vi "DecodePublicKey.vi"(3 "error in (no error) 2":errorcluster, 4 "Public Key":string) -> (0 "error out":errorcluster, 1 "e":cluster{"P/N":bool, "Array":u64[]}, 2 "n":cluster{"P/N":bool, "Array":u64[]})   [LabVIEW 2023]
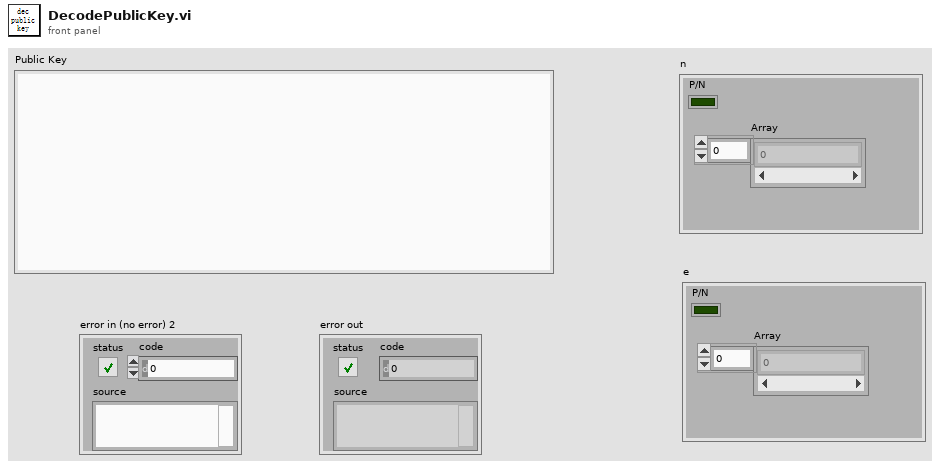
[diagram p1: front panel]
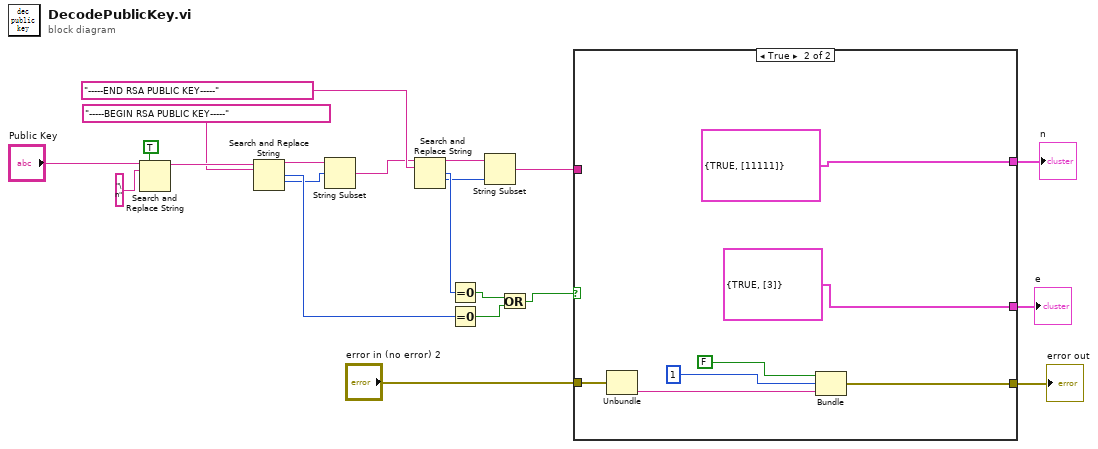
[diagram p0: block diagram]
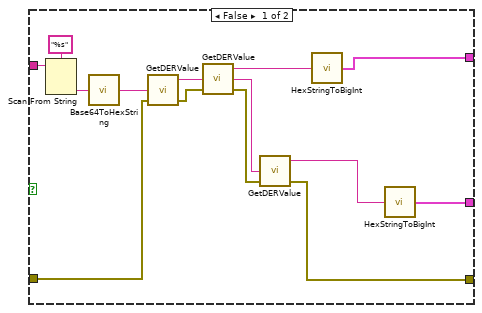
[diagram p2: hidden frame]
diagram:
  n1 = Search and Replace String(replace all?=TRUE, input string="Public Key", search string="\n") -> (result string=w18:string)  [unwired: 5 in, 3 out]
  n2 = Search and Replace String(input string=w18, search string="-----BEGIN RSA PUBLIC KEY-----") -> (result string=w13:string, number of replacements=w15:i32, offset past replacement=w12:i32)  [unwired: 6 in, 1 out]
  n3 = String Subset(string=w13, offset (0)=w12) -> (substring=w11:string)  [unwired: 1 in]
  n4 = Search and Replace String(input string=w11, search string="-----END RSA PUBLIC KEY-----") -> (result string=w10:string, number of replacements=w14:i32, offset past replacement=w9:i32)  [unwired: 6 in, 1 out]
  n5 = Equal To 0?(x=w14) -> (x = 0?=w7:bool)
  n6 = Equal To 0?(x=w15) -> (x = 0?=w6:bool)
  n7 = String Subset(string=w10, length (rest)=w9) -> (substring=w8:string)  [unwired: 1 in]
  n8 = Or(x=w7, y=w6) -> (x .or. y?=w5:bool)
  n9 = case shown="True" w5 {
    tunnel: w8 -> [w34 _]
    tunnel: [w29 cluster{bool, u64[]} {TRUE, [11111]}] -> w4
    tunnel: [w28 cluster{bool, u64[]} {TRUE, [3]}] -> w3
    tunnel: [w23 w36] -> w2
    tunnel: "error in (no error) 2" -> [w22 w40]
    frame False {
      n10 = Scan From String(format string="%s", input string=w34) -> (output 1=w33:string)  [unwired: 3 in, 3 out]
      n11 = call "Base64ToHexString.vi"("BASE64 string"=w33) -> ("Hex"=w31:string)
      n12 = call "GetDERValue.vi"("error in (no error)"=w22, "DER"=w31) -> ("error out"=w25:errorcluster, "value"=w30:string)  [unwired: 1 in, 1 out]
      n13 = call "GetDERValue.vi"("error in (no error)"=w25, "DER"=w30) -> ("error out"=w24:errorcluster, "remaining"=w32:string, "value"=w26:string)  [unwired: 1 in]
      n14 = call "GetDERValue.vi"("error in (no error)"=w24, "DER"=w32) -> ("error out"=w23:errorcluster, "value"=w27:string)  [unwired: 1 in, 1 out]
      n15 = call "HexStringToBigInt.vi"("String (hex)"=w26) -> ("Int"=w29:cluster{"P/N":bool, "Array":u64[]})
      n16 = call "HexStringToBigInt.vi"("String (hex)"=w27) -> ("Int"=w28:cluster{"P/N":bool, "Array":u64[]})
    }
    frame True {
      n17 = Unbundle(w40) -> ("source"=w39:string)  [unwired: 2 out]
      n18 = Bundle(FALSE, 1, "source"=w39) -> (w36:cluster{bool, i32, "source":string})  [unwired: 1 in]
    }
  }
  "n" <- w4
  "e" <- w3
  "error out" <- w2
